vi "Set Type.vi"(10 "Type":refnum<class "Type.lvclass">, 11 "RelationPanel in":refnum<class "RelationPanel.lvclass">) -> (3 "RelationPanel out":refnum<class "RelationPanel.lvclass">)   [LabVIEW 2020, in "Conditum-Tools.lvlib" / "RelationPanel.lvclass"]
uses:
  RelationPanel.lvclass
  Conditum-Clone/Columns/Type/Type.lvclass
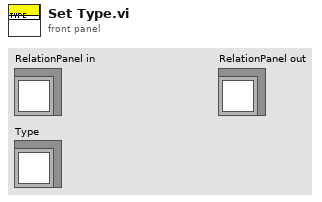
[diagram p1: front panel]
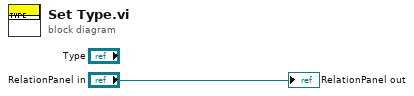
[diagram p0: block diagram]
diagram:
  "RelationPanel out" <- "RelationPanel in"
